vi "Show Settings UI.vi"(8 "Error In":errorcluster, 11 "Pane in":refnum<class "Pane.lvclass">) -> (0 "Error Out":errorcluster, 3 "Pane out":refnum<class "Pane.lvclass">)   [LabVIEW 2017, in "Pane.lvclass"]
uses:
  Pane.lvclass
  D:/software/LabView_PaneRelief_2017/test/D/software/LabView_PaneRelief_2017/Classes/Panel Object/Panel Object.lvclass
  Panel Object/Panel Object.lvclass/Panel Object.ctl
  Pane Settings UI/Pane Settings UI Messages/Show Pane Settings UI Msg/Show Pane Settings UI Msg.lvclass/Show Pane Settings UI Msg.ctl
  <vilib>/ActorFramework/Message Enqueuer/Message Enqueuer.lvclass/Message Enqueuer.ctl
  Panel Object/Read Settings UI Enqueuer.vi
  <vilib>/ActorFramework/Message Enqueuer/Enqueue.vi
  Pane Settings UI/Pane Settings UI Messages/Show Pane Settings UI Msg/Show Pane Settings UI Msg.lvclass
  C:/Program Files (x86)/National Instruments/LabVIEW 2017/vi.lib/ActorFramework/Message/Message.lvclass
  <vilib>/ActorFramework/Message Priority Queue/Priority Enqueue.vi
  <vilib>/ActorFramework/Message Enqueuer/Message Enqueuer.lvclass
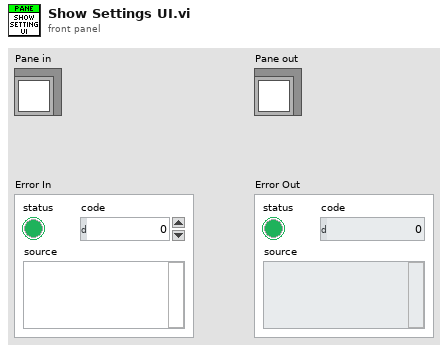
[diagram p1: front panel]
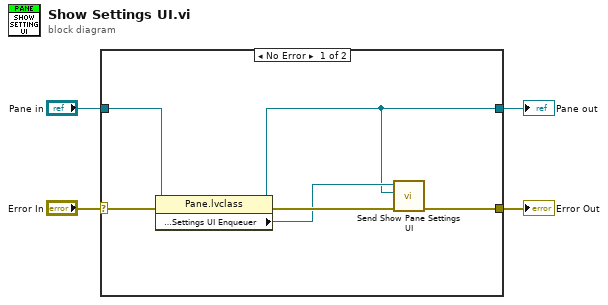
[diagram p0: block diagram]
diagram:
  n1 = case shown="No Error" "Error In" {
    selector: "Error In" -> [w10 w12]
    tunnel: [w7 w12] -> w1
    tunnel: [w5 w11] -> w3
    tunnel: "Pane in" -> [w9 w11]
    frame No Error {
      n2 = property class="Pane.lvclass"(reference=w9, error in=w10) -> (reference out=w5:refnum<class "Pane.lvclass">, error out=w8:errorcluster, "Protected Accessors:Settings UI Enqueuer"=w6:refnum<class "Message Enqueuer.lvclass">)
      n3 = call "Send Show Pane Settings UI.vi"("error in (no error)"=w8, "Pane"=w5, "Message Enqueuer"=w6) -> ("error out"=w7:errorcluster)  [unwired: 7 in, 1 out]
    }
    frame Error {
    }
  }
  "Pane out" <- w3
  "Error Out" <- w1
